vi "NP_Logging_libESP301.vi"(0 "Instrument Channel":string="GPIB/0:4,0", 1 "Prefix (Instrument name)":string, 2 "String 1 Enable (T)":bool=TRUE, 3 "Generic Strings":bool, 5 "String 1 {Write} (in)":string, 7 "String 2 {Read} (in)":string, 9 "Filename (Data.log)":string="Data.log", 11 "error in (no error)":errorcluster, 12 "Operating Mode (Logging)":T1=enum."Logging", 13 "String 2 Enable (T)":bool=TRUE) -> (4 "Instrument Channel out":string="GPIB/0:4,0", 6 "String 1 {Write} (out)":string, 8 "String 2 {Read} (out)":string, 15 "error out":errorcluster)   [LabVIEW 2019, in "Newport ESP301.lvlib"]
doc: "This VI will enable logging of communication to a text file.\n\nIt will put timestamp and strings in the log file. \n\nIt can be used for Query/Response, or Generically for any logging.\nThe Label will be after the timestamp.\n\nNormal Operating Mode will disable logging."
uses:
  Newport ESP301.lvlib
  ctl_OperatingMode_libESP301.ctl
panel:
  in  "Show Interval":bool
  # "If Generic then Prefix will not indicate Write and Response."
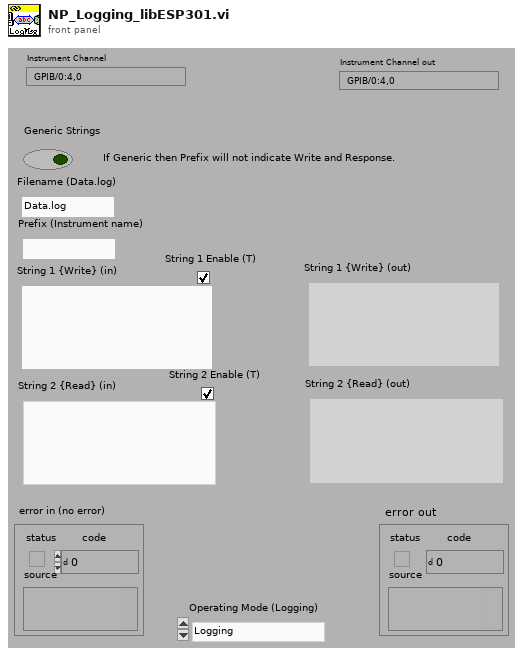
[diagram p1: front panel]
types:
  T1 = typedef "Newport ESP301.lvlib/ctl_OperatingMode_libESP301.ctl" = enum16{"Normal", "Logging", "Simulation w/Zeroes", "Simulation from Log File"}
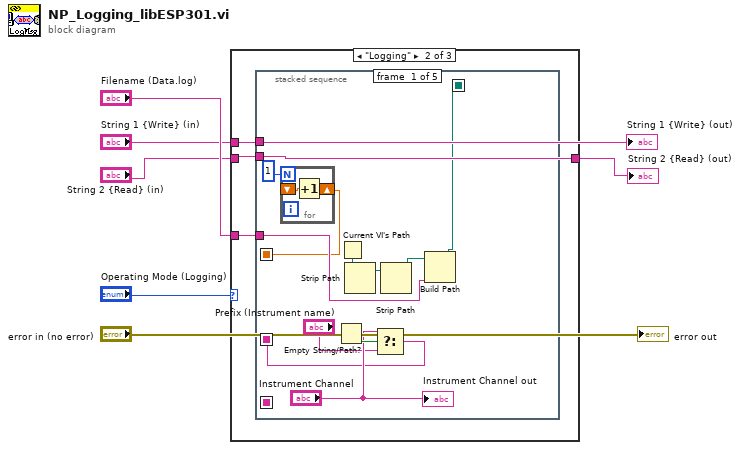
[diagram p0: block diagram]
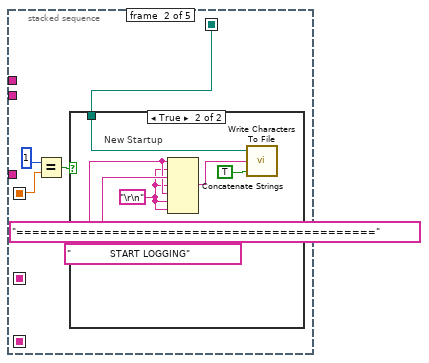
[diagram p3: hidden frame]
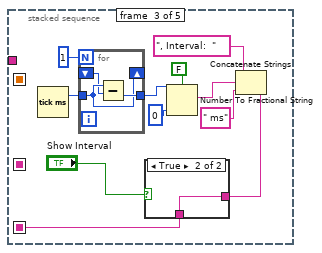
[diagram p5: hidden frame]
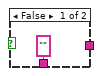
[diagram p6: hidden frame]
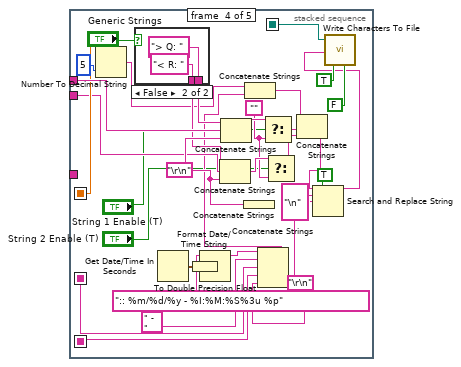
[diagram p7: hidden frame]
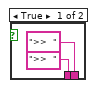
[diagram p8: hidden frame]
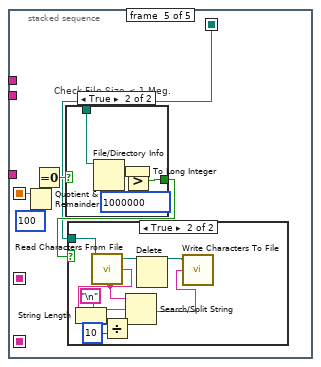
[diagram p9: hidden frame]
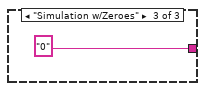
[diagram p12: hidden frame]
diagram:
  n1 = case shown="\"Logging\"" "Operating Mode (Logging)" {
    tunnel: "String 1 {Write} (in)" -> [_ w9 _]
    tunnel: "String 2 {Read} (in)" -> [w7 w10 _]
    tunnel: [w7 w10 "0"] -> w5
    tunnel: "Filename (Data.log)" -> [_ w8 _]
    frame "Normal", Default {
    }
    frame "Logging" {
      n2 = stacked-sequence {
        seq-local: [w15 _ _ _ _] -> [_ w26 _ w76 w90]
        seq-local: [w16 _ _ _ _] -> [_ w24 _ w75 w87]
        seq-local: [w11 _ _ _ _] -> [_ _ _ w57 _]
        seq-local: [_ _ w34 _ _] -> [_ _ _ w52 _]
        tunnel: w10 -> [_ _ _ w71 _]
        tunnel: w9 -> [_ _ _ w80 _]
        tunnel: w8 -> [w18 _ _ _ _]
        frame #0 {
          n3 = for {
            N: 1 -> [_]
            shift-right: [w22] -> w15
            shift-left: _ -> [w23]
            n4 = Increment(x=w23) -> (x+1=w22:dbl)
          }
          n5 = Empty String/Path?(string/path="Prefix (Instrument name)") -> (empty?=w14:bool)
          n6 = Current VI's Path() -> (path=w21:path)
          n7 = Strip Path(path=w21) -> (stripped path=w20:path)  [unwired: 1 out]
          n8 = Select(t="Instrument Channel", s=w14, f="Prefix (Instrument name)") -> (s? t:f=w11:string)
          n9 = Strip Path(path=w20) -> (stripped path=w19:path)  [unwired: 1 out]
          n10 = Build Path(base path=w19, name or relative path=w18) -> (appended path=w16:path)
          "Instrument Channel out" <- "Instrument Channel"
        }
        frame #1 {
          n11 = Equal?(x=1, y=w26) -> (x = y?=w25:bool)
          n12 = case shown="True" w25 {
            tunnel: w24 -> [_ w33]
            frame False {
            }
            frame True {
              w29 = "\r\n"
              w30 = "============================================="
              # "New Startup"
              n13 = Concatenate Strings(w30, w29, "             START LOGGING", w29, w30, w29, w29) -> (w28:string)
              n14 = call <vilib>:"Write Characters To File.vi"("append to file? (new file:F)"=TRUE, "character string"=w28, "file path (dialog if empty)"=w33) -> ()  [unwired: 2 in, 1 out]
            }
          }
        }
        frame #2 {
          n15 = Tick Count (ms)() -> (millisecond timer value=w44:u32)
          n16 = for {
            N: 1 -> [_]
            shift-right: [w48] -> _
            shift-left: _ -> [w47]
            tunnel: w44 -> [w48]
            tunnel: [w49] -> w42
            n17 = Subtract(x=w48, y=w47) -> (x-y=w49:u32)
          }
          n18 = Number To Fractional String(use system decimal point (T)=FALSE, number=w42, precision (6)=i16 0) -> (F-format string=w39:string)  [unwired: 1 in]
          n19 = Concatenate Strings(", Interval:  ", w39, " ms") -> (w35:string)
          n20 = case shown="True" "Show Interval" {
            tunnel: w35 -> [_ w46]
            tunnel: ["" w46] -> w34
            frame False {
            }
            frame True {
            }
          }
        }
        frame #3 {
          w62 = ""
          w72 = "\r\n"
          w51 = "\r\n"
          n21 = Number To Decimal String(number=w76, width (-)=i16 5) -> (decimal integer string=w69:string)
          n22 = case shown="False" "Generic Strings" {
            tunnel: [">>  " "< R: "] -> w70
            tunnel: [">>  " "> Q: "] -> w74
            frame True {
            }
            frame False {
            }
          }
          n23 = Get Date/Time In Seconds() -> (seconds since 1Jan1904=w50:timestamp)
          n24 = To Double Precision Float(number=w50) -> (double precision float=w79:dbl)
          n25 = Format Date/Time String(time format string (%c)=":: %m/%d/%y - %I:%M:%S%3u %p", seconds (now)=w79) -> (date/time string=w59:string)  [unwired: 1 in]
          n26 = Concatenate Strings(w70, w71, w72) -> (w66:string)
          n27 = Concatenate Strings(w74, w80, w72) -> (w64:string)
          n28 = Concatenate Strings(w72) -> ()  [unwired: 1 out]
          n29 = Concatenate Strings(w59, " - ", w57, w52, w51) -> (w68:string)
          n30 = Concatenate Strings(w69, w68) -> (w67:string)
          n31 = Select(t=w64, s="String 1 Enable (T)", f=w62) -> (s? t:f=w65:string)
          n32 = Select(t=w66, s="String 2 Enable (T)", f=w62) -> (s? t:f=w63:string)
          n33 = Concatenate Strings(w67, w65, w63) -> (w56:string)
          n34 = Search and Replace String(replace all?=TRUE ("replace all? (F)"), input string=w56, search string="\n", replace string=w51) -> (result string=w53:string)  [unwired: 4 in, 3 out]
          n35 = call <vilib>:"Write Characters To File.vi"("convert eol? (no:F)"=FALSE, "append to file? (new file:F)"=TRUE, "character string"=w53, "file path (dialog if empty)"=w75) -> ()  [unwired: 1 in, 1 out]
        }
        frame #4 {
          # "Check File Size < 1 Meg."
          n36 = Quotient & Remainder(x=w90, y=100) -> (x-y*floor(x/y)=w91:i32)  [unwired: 1 out]
          n37 = Equal To 0?(x=w91) -> (x = 0?=w89:bool)
          n38 = case shown="True" w89 {
            selector: w89 -> [w102 _]
            tunnel: w87 -> [_ w107]
            tunnel: [w102 w104] -> w88
            frame False {
            }
            frame True {
              n39 = File/Directory Info(path=w107) -> (size=w103:i64)  [unwired: 1 in, 6 out]
              n40 = To Long Integer(number=w103) -> (32bit integer=w106:i32)
              n41 = Greater?(x=w106, y=1000000) -> (0:w104:bool)
            }
          }
          n42 = case shown="True" w88 {
            tunnel: w87 -> [_ w101]
            frame False {
            }
            frame True {
              n43 = call <vilib>:"Read Characters From File.vi"("file path (dialog if empty)"=w101) -> ("new file path (NotAPath if cancelled)"=w94:path, "character string"=w99:string)  [unwired: 5 in, 2 out]
              n44 = String Length(string=w99) -> (length=w98:i32)
              n45 = Divide(x=w98, y=10) -> (x/y=w96:dbl)
              n46 = Search/Split String(string=w99, search string/char (-)="\n", offset (0)=w96) -> (match + rest of string=w95:string)  [unwired: 2 out]
              n47 = Delete(path (use dialog)=w94) -> (deleted path=w93:path)  [unwired: 4 in, 2 out]
              n48 = call <vilib>:"Write Characters To File.vi"("character string"=w95, "file path (dialog if empty)"=w93) -> ()  [unwired: 3 in, 1 out]
            }
          }
        }
      }
    }
    frame "Simulation w/Zeroes" {
    }
  }
  "String 2 {Read} (out)" <- w5
  "error out" <- "error in (no error)"
  "String 1 {Write} (out)" <- "String 1 {Write} (in)"
